vi "Dac_Output_cam_trig_multiple_digital_signals_synchronized.vi"(0 "File to read":path=path "C:/Users/lpk27/Documents/pan-ASLMsynched/pan-ASLM/Calibration files/newcalibration_voice coil input_25msflyback.txt", 1 "Image acquisition time (ms)":dbl=1000.0, 2 "Delay between frames (ms)":dbl=25.0, 3 "typedef_laser_order_control":T1={"Laser 560 nm order selection"=0, "Laser 595 nm order selection"=0, "Laser 642 nm order selection"=0, "Laser 488 nm order selection"=1, "Color Box"=60927, "Color Box 2"=12844800, "Color Box 3"=14132992, "Color Box 4"=16715008} {"Laser 488 nm order selection" items=["Not active", "1", "2", "3", "4"]; "Laser 642 nm order selection" items=["Not active", "1", "2", "3", "4"]; "Laser 595 nm order selection" items=["Not active", "1", "2", "3", "4"]; "Laser 560 nm order selection" items=["Not active", "1", "2", "3", "4"]}, 4 "stop":bool, 5 "error in":errorcluster, 6 "Number of slices":i32=1000, 7 "Camera trigger initial delay [ms]":dbl format="%.6f", 11 "Setup":enum16{"Test setup", "Microscope"}(ring)) -> (19 "error out":errorcluster)   [LabVIEW 2020]
uses:
  typedefs/typedef_laser_order_control.ctl
  <vilib>/DAQmx/write.llb/DAQmx Write (Digital Wfm 1Chan NSamp).vi
  <vilib>/DAQmx/write.llb/DAQmx Write (Analog Wfm 1Chan NSamp).vi
  <vilib>/Utility/file.llb/Read Delimited Spreadsheet (DBL).vi
  <vilib>/DAQmx/create/channels.llb/DAQmx Create Channel (AO-Voltage-Basic).vi
  <vilib>/DAQmx/configure/timing.llb/DAQmx Timing (Sample Clock).vi
  <vilib>/DAQmx/miscellaneous.llb/DAQmx Fill In Error Info.vi
  Global stop DAQ.vi
  <vilib>/DAQmx/create/channels.llb/DAQmx Create Channel (CO-Pulse Generation-Ticks).vi
  <vilib>/DAQmx/configure/timing.llb/DAQmx Timing (Implicit).vi
  <vilib>/DAQmx/create/channels.llb/DAQmx Create Channel (DO-Digital Output).vi
  <vilib>/Waveform/DWDTOps.llb/DWDT Uncompress Digital.vi
  <vilib>/DAQmx/create/channels.llb/DAQmx Create Channel (CO-Pulse Generation-Frequency).vi
  <vilib>/DAQmx/configure/trigger.llb/DAQmx Start Trigger (Digital Edge).vi
  Global DAQ started.vi
  Global Counter count.vi
  <resource>/objmgr/daqmx.rc
panel:
  out "CO.Count":u32
  out "error out 4":errorcluster
  out "error out 3":errorcluster
  out "error out 2":errorcluster
  out "Digital Waveform Graph":digitalwaveform(graph)
  out "LabVIEW generated Sawtooth input (blue) and Camera trigger (red)":waveform(dbl)(graph)={"t0"=timestamp(0 s since 1904-01-01), "dt"=1.0, "Y"=array[3075 elements]}
  out "# Samples written per channel":u32=3075
  out "actual frequency":dbl=1000.0
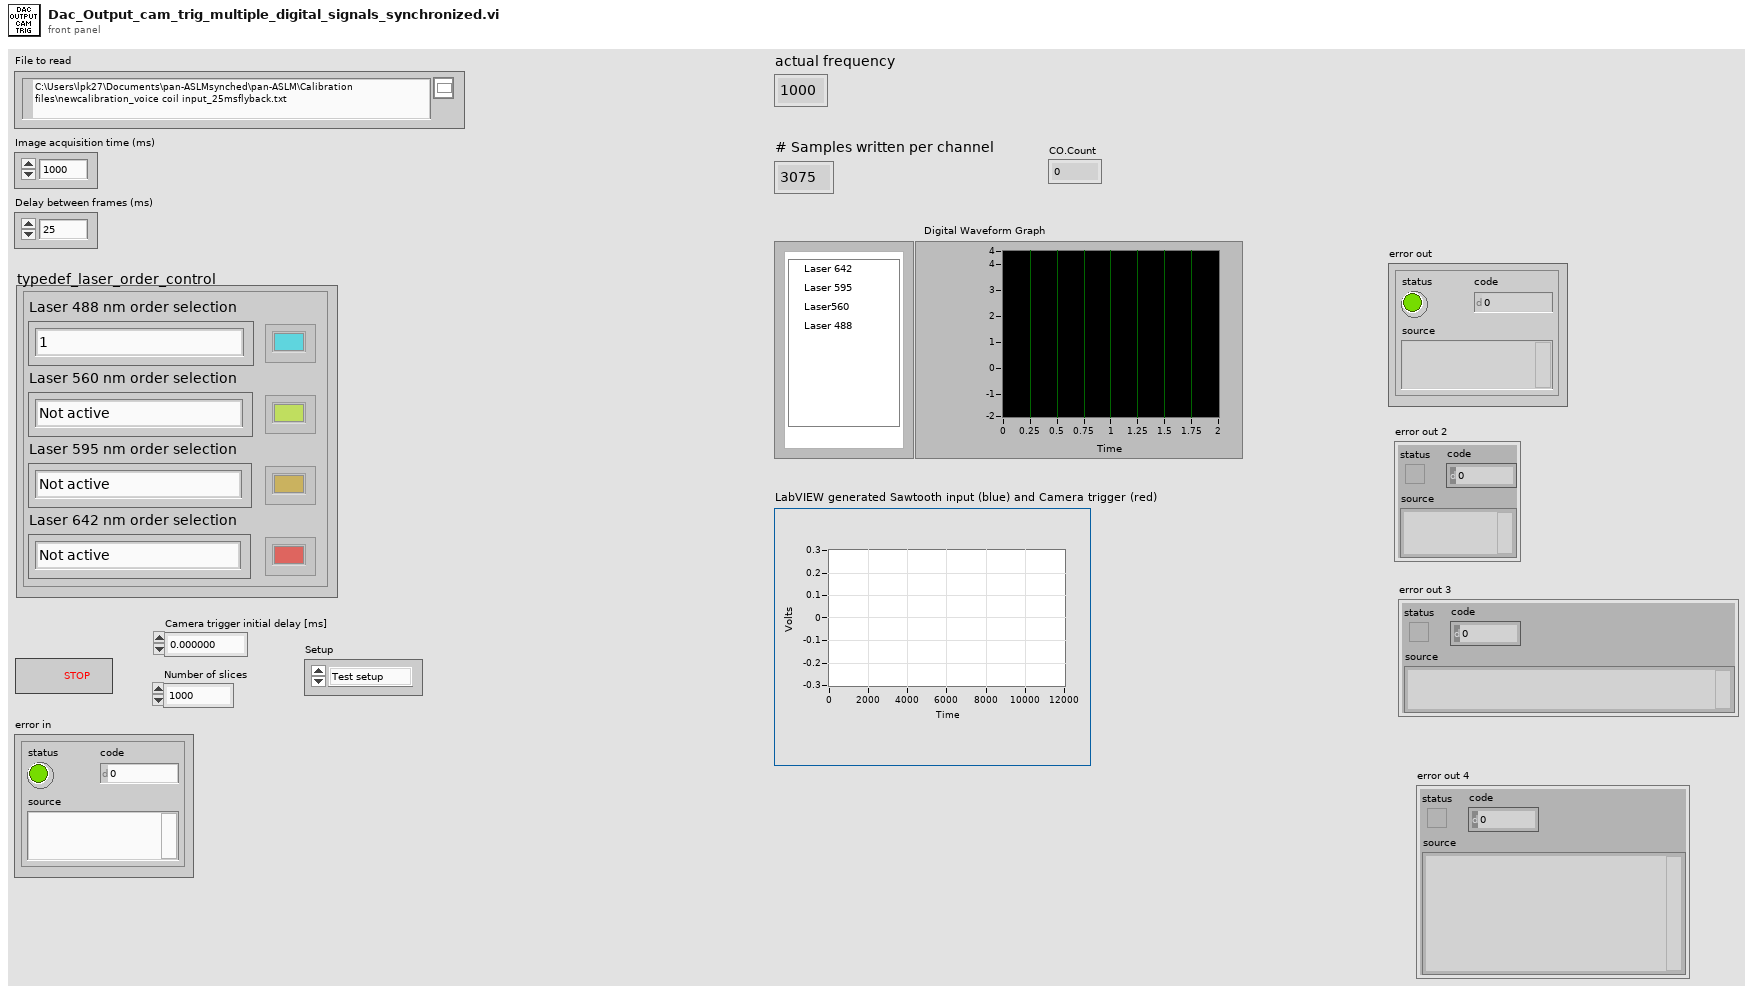
[diagram p1: front panel]
types:
  T1 = typedef "typedef_laser_order_control.ctl" = cluster{"Laser 560 nm order selection":u16, "Laser 595 nm order selection":u16, "Laser 642 nm order selection":u16, "Laser 488 nm order selection":u16, "Color Box":u32, "Color Box 2":u32, "Color Box 3":u32, "Color Box 4":u32}
  T2 = typedef "DAQ_channel_typedef.ctl" = cluster{"CO.Pulse.Term":tag, "Voice coil analog output":tag, "counter":tag, "CO.Pulse.Term 2":tag, "AOTF lines":tag, "counter 2":tag, "CO.Pulse.Term 3":tag, "counter 3":tag}
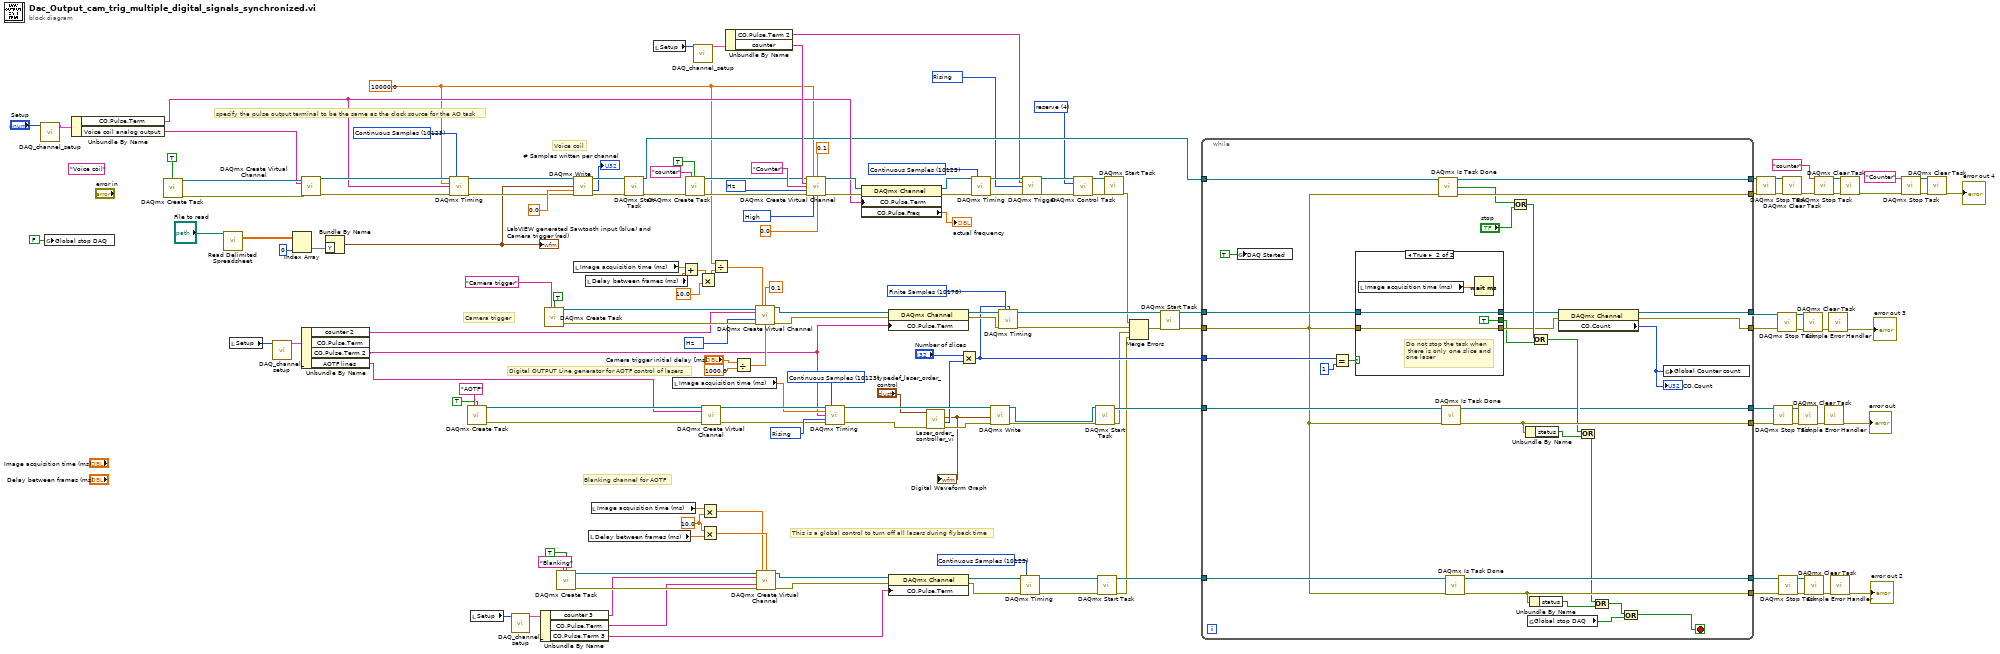
[diagram p0: block diagram]
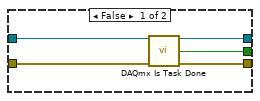
[diagram p2: hidden frame]
diagram:
  w2 = 10123 items=["Finite Samples"=10178, "Continuous Samples"=10123, "Hardware Timed Single Point"=12522] ("sample mode")
  w10 = 10.0 ("y")
  w22 = 4 items=["verify"=2, "reserve"=4, "commit"=3, "unreserve"=5, "abort"=6] ("action")
  w26 = 10280 items=["Rising"=10280, "Falling"=10171] ("edge")
  w43 = 10373 items=["Hz"=10373] ("units")
  (unwired) "Voice coil" ("new task name")
  w120 = 10123 items=["Finite Samples"=10178, "Continuous Samples"=10123, "Hardware Timed Single Point"=12522] ("sample mode")
  w125 = 10280 items=["Rising"=10280, "Falling"=10171] ("active edge")
  w134 = 10178 items=["Finite Samples"=10178, "Continuous Samples"=10123, "Hardware Timed Single Point"=12522] ("sample mode")
  w145 = 10192 items=["High"=10192, "Low"=10214] ("idle state")
  w146 = 10373 items=["Hz"=10373] ("units")
  w139 = 10123 items=["Finite Samples"=10178, "Continuous Samples"=10123, "Hardware Timed Single Point"=12522] ("sample mode")
  w42 = 10000.0 ("rate")
  w156 = 10123 items=["Finite Samples"=10178, "Continuous Samples"=10123, "Hardware Timed Single Point"=12522] ("sample mode")
  # "This is a global control to turn off all lasers during flyback time"
  # "Voice coil"
  # "Camera trigger"
  # "Digital OUTPUT Line generator for AOTF control of lasers"
  # "Blanking channel for AOTF"
  # "specify the pulse output terminal to be the same as the clock source for the AO task"
  n1 = call "DAQ_channel_setup.vi"("Text Ring"="Setup") -> ("DAQ channels OUT"=w68:T2)  [unwired: 10 in]
  n2 = global write "Global stop DAQ.vi" "Global stop DAQ"(FALSE ("Global stop DAQ")) -> ()
  n3 = Unbundle By Name(w68) -> ("CO.Pulse.Term"=w48:tag, "Voice coil analog output"=w69:tag)
  n4 = call <vilib>:"DAQmx Create Task.vi"("auto cleanup"=TRUE) -> ("task out"=w105:refnum<k21>, "error out"=w104:errorcluster)  [unwired: 13 in]
  n5 = call-poly <vilib>:"Read Delimited Spreadsheet.vi"("file path (dialog if empty)"="File to read") -> ("all rows"=w131:dbl[][])  [unwired: 9 in, 5 out]
  n6 = local read "Setup"() -> (w57:enum16{"Test setup", "Microscope"})
  n7 = call "DAQ_channel_setup.vi"("Text Ring"=w57) -> ("DAQ channels OUT"=w65:T2)  [unwired: 10 in]
  n8 = Index Array(array=w131, index (col)=0 ("disabled index (col)")) -> (element=w129:dbl[])  [unwired: 1 in]
  n9 = call-poly <vilib>:"DAQmx Create Virtual Channel.vi"("task in"=w105, "physical channels"=w69, "error in"=w104) -> ("task out"=w158:refnum<k21>, "error out"=w157:errorcluster)  [unwired: 11 in]
  n10 = Unbundle By Name(w65) -> ("counter 2"=w60:tag, "CO.Pulse.Term 2"=w14:tag, "AOTF lines"=w64:tag)  [unwired: 1 out]
  n11 = Bundle By Name("Y"=w129) -> (w128:waveform(dbl))  [unwired: 1 in]
  "LabVIEW generated Sawtooth input (blue) and Camera trigger (red)" <- w128
  n12 = call-poly <vilib>:"DAQmx Timing.vi"("task/channels in"=w158, "sample mode"=w156, "rate"=w42, "source"=w48, "error in"=w157) -> ("task out"=w141:refnum<k21>, "error out"=w140:errorcluster)  [unwired: 9 in]
  n13 = call <vilib>:"DAQmx Create Task.vi"("new task name"="AOTF", "auto cleanup"=TRUE) -> ("task out"=w107:refnum<k21>, "error out"=w106:errorcluster)  [unwired: 12 in]
  n14 = local read "Setup"() -> (w58:enum16{"Test setup", "Microscope"})
  n15 = call "DAQ_channel_setup.vi"("Text Ring"=w58) -> ("DAQ channels OUT"=w63:T2)  [unwired: 10 in]
  n16 = Unbundle By Name(w63) -> ("counter 3"=w62:tag, "CO.Pulse.Term"=w1:tag, "CO.Pulse.Term 3"=w61:tag)
  n17 = call <vilib>:"DAQmx Create Task.vi"("new task name"="Camera trigger", "auto cleanup"=TRUE) -> ("task out"=w102:refnum<k21>, "error out"=w103:errorcluster)  [unwired: 12 in]
  n18 = call <vilib>:"DAQmx Create Task.vi"("new task name"="Blanking", "auto cleanup"=TRUE) -> ("task out"=w110:refnum<k21>, "error out"=w109:errorcluster)  [unwired: 12 in]
  n19 = call-poly <vilib>:"DAQmx Write.vi"("task/channels in"=w141, "data"=w128, "timeout"=0.0, "error in"=w140) -> ("task out"=w150:refnum<k21>, "number of samples written per channel"=→"# Samples written per channel":u32, "error out"=w149:errorcluster)  [unwired: 9 in]
  n20 = local read "Image acquisition time (ms)"() -> (w113:dbl)
  n21 = local read "Delay between frames (ms)"() -> (w112:dbl)
  n22 = local read "Delay between frames (ms)"() -> (w9:dbl)
  n23 = local read "Image acquisition time (ms)"() -> (w12:dbl)
  n24 = call <vilib>:"DAQmx Start Task.vi"("task/channels in"=w150, "error in"=w149) -> ("task out"=w47:refnum<k21>, "error out"=w144:errorcluster)  [unwired: 12 in]
  n25 = local read "Setup"() -> (w56:enum16{"Test setup", "Microscope"})
  n26 = local read "Image acquisition time (ms)"() -> (w116:dbl)
  n27 = Add(x=w113, y=w112) -> (x+y=w34:dbl)
  n28 = call <vilib>:"DAQmx Create Task.vi"("new task name"="counter", "auto cleanup"=TRUE, "error in"=w144) -> ("task out"=w53:refnum<k21>, "error out"=w155:errorcluster)  [unwired: 11 in]
  n29 = call "DAQ_channel_setup.vi"("Text Ring"=w56) -> ("DAQ channels OUT"=w67:T2)  [unwired: 10 in]
  n30 = Multiply(x=w34, y=10.0) -> (x*y=w33:dbl)
  n31 = Multiply(x=w12, y=w10) -> (x*y=w11:dbl)
  n32 = Multiply(x=w10, y=w9) -> (x*y=w13:dbl)
  n33 = call-poly <vilib>:"DAQmx Create Virtual Channel.vi"("task in"=w107, "lines"=w64, "error in"=w106) -> ("task out"=w124:refnum<k21>, "error out"=w123:errorcluster)  [unwired: 11 in]
  n34 = Divide(x=w42, y=w33) -> (x/y=w45:dbl)
  n35 = Unbundle By Name(w67) -> ("CO.Pulse.Term 2"=w25:tag, "counter"=w66:tag)
  n36 = Divide(x="Camera trigger initial delay [ms]", y=1000.0) -> (x/y=w29:dbl)
  n37 = call-poly <vilib>:"DAQmx Create Virtual Channel.vi"("task in"=w102, "frequency"=w45, "duty cycle"=0.1, "counter"=w60, "units"=w43, "error in"=w103, "initial delay"=w29) -> ("task out"=w138:refnum<k21>, "error out"=w127:errorcluster)  [unwired: 7 in]
  n38 = call-poly <vilib>:"DAQmx Create Virtual Channel.vi"("task in"=w110, "high ticks"=w11, "low ticks"=w13, "counter"=w62, "source of ticks"=w1, "error in"=w109) -> ("task out"=w119:refnum<k21>, "error out"=w117:errorcluster)  [unwired: 8 in]
  n39 = call-poly <vilib>:"DAQmx Create Virtual Channel.vi"("task in"=w53, "frequency"=w42, "duty cycle"=0.1, "counter"=w66, "name to assign"="Counter", "units"=w146, "error in"=w155, "idle state"=w145, "initial delay"=0.0) -> ("task out"=w154:refnum<k21>, "error out"=w153:errorcluster)  [unwired: 5 in]
  n40 = call-poly <vilib>:"DAQmx Timing.vi"("task/channels in"=w124, "sample mode"=w120, "rate"=w116, "source"=w14, "active edge"=w125, "error in"=w123) -> ("task out"=w122:refnum<k21>, "error out"=w115:errorcluster)  [unwired: 8 in]
  n41 = property class="DAQmx Channel"(reference=w154, error in=w153, "CO.Pulse.Term"=w48) -> (reference out=w151:refnum<k21>, error out=w152:errorcluster, "CO.Pulse.Freq"=→"actual frequency":dbl)
  n42 = property class="DAQmx Channel"(reference=w138, error in=w127, "CO.Pulse.Term"=w14) -> (reference out=w126:refnum<k21>, error out=w135:errorcluster)
  n43 = property class="DAQmx Channel"(reference=w119, error in=w117, "CO.Pulse.Term"=w61) -> (reference out=w6:refnum<k21>, error out=w5:errorcluster)
  n44 = call "Laser_order_controller_vi.vi"("error in"=w115, "typedef_laser_order_control"="typedef_laser_order_control") -> ("error out"=w114:errorcluster, "Active lasers"=w38:i16, "Digital Waveform Graph"=w37:digitalwaveform)  [unwired: 7 in]
  "Digital Waveform Graph" <- w37
  n45 = Multiply(x="Number of slices", y=w38) -> (x*y=w36:i32)
  n46 = call-poly <vilib>:"DAQmx Timing.vi"("task/channels in"=w151, "sample mode"=w139, "error in"=w152) -> ("task out"=w28:refnum<k21>, "error out"=w27:errorcluster)  [unwired: 11 in]
  n47 = call-poly <vilib>:"DAQmx Write.vi"("task/channels in"=w122, "data"=w37, "error in"=w114) -> ("task out"=w7:refnum<k21>, "error out"=w8:errorcluster)  [unwired: 10 in, 1 out]
  n48 = call-poly <vilib>:"DAQmx Timing.vi"("task/channels in"=w126, "sample mode"=w134, "samples per channel"=w36, "error in"=w135) -> ("task out"=w133:refnum<k21>, "error out"=w17:errorcluster)  [unwired: 10 in]
  n49 = call-poly <vilib>:"DAQmx Timing.vi"("task/channels in"=w6, "sample mode"=w2, "error in"=w5) -> ("task out"=w4:refnum<k21>, "error out"=w3:errorcluster)  [unwired: 11 in]
  n50 = call-poly <vilib>:"DAQmx Trigger.vi"("task/channels in"=w28, "source"=w25, "edge"=w26, "error in"=w27) -> ("task out"=w24:refnum<k21>, "error out"=w23:errorcluster)  [unwired: 10 in]
  n51 = call <vilib>:"DAQmx Control Task.vi"("task/channels in"=w24, "action"=w22, "error in"=w23) -> ("task out"=w21:refnum<k21>, "error out"=w20:errorcluster)  [unwired: 11 in]
  n52 = call <vilib>:"DAQmx Start Task.vi"("task/channels in"=w7, "error in"=w8) -> ("task out"=w121:refnum<k21>, "error out"=w16:errorcluster)  [unwired: 12 in]
  n53 = call <vilib>:"DAQmx Start Task.vi"("task/channels in"=w4, "error in"=w3) -> ("task out"=w118:refnum<k21>, "error out"=w15:errorcluster)  [unwired: 12 in]
  n54 = call <vilib>:"DAQmx Start Task.vi"("task/channels in"=w21, "error in"=w20) -> ("error out"=w18:errorcluster)  [unwired: 12 in, 1 out]
  n55 = Merge Errors(w18, w17, w16, w15) -> (w19:errorcluster)
  n56 = call <vilib>:"DAQmx Start Task.vi"("task/channels in"=w133, "error in"=w19) -> ("task out"=w137:refnum<k21>, "error out"=w136:errorcluster)  [unwired: 12 in]
  n57 = while {
    tunnel: w47 -> [w189]
    tunnel: w137 -> [w188]
    tunnel: w136 -> [w159]
    tunnel: w121 -> [w187]
    tunnel: w118 -> [w186]
    tunnel: [w185] -> w87
    tunnel: [w179] -> w86
    tunnel: [w169] -> w92
    tunnel: [w167] -> w91
    tunnel: [w171] -> w81
    tunnel: [w184] -> w80
    tunnel: [w183] -> w79
    tunnel: [w182] -> w78
    tunnel: w36 -> [w163]
    stop <- w164 stop-if-true
    n58 = global write "Global DAQ started.vi" "DAQ Started"(TRUE ("DAQ Started")) -> ()
    n59 = Equal?(x=w163, y=1) -> (x = y?=w161:bool)
    n60 = case shown="True" w161 {
      tunnel: w188 -> [w194 w198]
      tunnel: w159 -> [w193 w197]
      tunnel: [w192 w198] -> w170
      tunnel: [w191 w197] -> w168
      tunnel: [w190 TRUE ("task done?")] -> w165
      frame False {
        n61 = call <vilib>:"DAQmx Is Task Done.vi"("task/channels in"=w194, "error in"=w193) -> ("task out"=w192:refnum<k21>, "task done?"=w190:bool, "error out"=w191:errorcluster)  [unwired: 11 in]
      }
      frame True {
        # "Do not stop the task when\n there is only one slice and \none laser"
        n62 = local read "Image acquisition time (ms)"() -> (w195:dbl)
        n63 = Wait (ms)(milliseconds to wait=w195) -> ()  [unwired: 1 out]
      }
    }
    n64 = call <vilib>:"DAQmx Is Task Done.vi"("task/channels in"=w189, "error in"=w159) -> ("task out"=w185:refnum<k21>, "task done?"=w160:bool, "error out"=w179:errorcluster)  [unwired: 11 in]
    n65 = call <vilib>:"DAQmx Is Task Done.vi"("task/channels in"=w187, "error in"=w159) -> ("task out"=w171:refnum<k21>, "error out"=w184:errorcluster)  [unwired: 11 in, 1 out]
    n66 = call <vilib>:"DAQmx Is Task Done.vi"("task/channels in"=w186, "error in"=w159) -> ("task out"=w183:refnum<k21>, "error out"=w182:errorcluster)  [unwired: 11 in, 1 out]
    n67 = Or(x=w160, y="stop") -> (x .or. y?=w173:bool)
    n68 = Unbundle By Name(w184) -> ("status"=w178:bool)
    n69 = global read "Global stop DAQ.vi" "Global stop DAQ"() -> (w175:bool)
    n70 = Unbundle By Name(w182) -> ("status"=w176:bool)
    n71 = Or(x=w173, y=w165) -> (x .or. y?=w181:bool)
    n72 = property class="DAQmx Channel"(reference=w170, error in=w168) -> (reference out=w169:refnum<k21>, error out=w167:errorcluster, "CO.Count"=w166:u32)
    "CO.Count" <- w166
    n73 = Or(x=w181, y=w178) -> (x .or. y?=w180:bool)
    n74 = Or(x=w180, y=w176) -> (x .or. y?=w177:bool)
    n75 = Or(x=w177, y=w175) -> (x .or. y?=w164:bool)
    n76 = global write "Global Counter count.vi" "Global Counter count"(w166) -> ()
  }
  n77 = call <vilib>:"DAQmx Stop Task.vi"("task/channels in"=w87, "error in"=w86) -> ("task out"=w90:refnum<k21>, "error out"=w89:errorcluster)  [unwired: 12 in]
  n78 = call <vilib>:"DAQmx Stop Task.vi"("task/channels in"=w81, "error in"=w80) -> ("task out"=w84:refnum<k21>, "error out"=w85:errorcluster)  [unwired: 12 in]
  n79 = call <vilib>:"DAQmx Stop Task.vi"("task/channels in"=w92, "error in"=w91) -> ("task out"=w95:refnum<k21>, "error out"=w96:errorcluster)  [unwired: 12 in]
  n80 = call <vilib>:"DAQmx Stop Task.vi"("task/channels in"=w79, "error in"=w78) -> ("task out"=w76:refnum<k21>, "error out"=w77:errorcluster)  [unwired: 12 in]
  n81 = call <vilib>:"DAQmx Clear Task.vi"("task in"=w90, "error in"=w89) -> ("error out"=w71:errorcluster)  [unwired: 13 in]
  n82 = call <vilib>:"DAQmx Clear Task.vi"("task in"=w84, "error in"=w85) -> ("error out"=w83:errorcluster)  [unwired: 13 in]
  n83 = call <vilib>:"DAQmx Clear Task.vi"("task in"=w95, "error in"=w96) -> ("error out"=w94:errorcluster)  [unwired: 13 in]
  n84 = call <vilib>:"DAQmx Clear Task.vi"("task in"=w76, "error in"=w77) -> ("error out"=w75:errorcluster)  [unwired: 13 in]
  n85 = call <vilib>:"DAQmx Stop Task.vi"("task/channels in"="counter" ("new task name"), "error in"=w71) -> ("task out"=w73:refnum<k21>, "error out"=w72:errorcluster)  [unwired: 12 in]
  n86 = call <vilib>:"Simple Error Handler.vi"("error in (no error)"=w83) -> ("error out"=→"error out":errorcluster)  [unwired: 4 in, 4 out]
  n87 = call <vilib>:"Simple Error Handler.vi"("error in (no error)"=w94) -> ("error out"=→"error out 3":errorcluster)  [unwired: 4 in, 4 out]
  n88 = call <vilib>:"Simple Error Handler.vi"("error in (no error)"=w75) -> ("error out"=→"error out 2":errorcluster)  [unwired: 4 in, 4 out]
  n89 = call <vilib>:"DAQmx Clear Task.vi"("task in"=w73, "error in"=w72) -> ("error out"=w70:errorcluster)  [unwired: 13 in]
  n90 = call <vilib>:"DAQmx Stop Task.vi"("task/channels in"="Counter" ("new task name"), "error in"=w70) -> ("task out"=w50:refnum<k21>, "error out"=w51:errorcluster)  [unwired: 12 in]
  n91 = call <vilib>:"DAQmx Clear Task.vi"("task in"=w50, "error in"=w51) -> ("error out"=→"error out 4":errorcluster)  [unwired: 13 in]
